vi "Two Camera.vi"() -> ()   [LabVIEW 2015]
uses:
  <vilib>/userdefined/High Color/IMAQdx.ctl
  <vilib>/vision/driver/NI_Vision_Acquisition_Software.lvlib
panel:
  in  "Save":bool
  in  "Session In 2":T1
  in  "Session In":T1
  out "Image 2":T2(plugin-control)
  out "Frame Rate 2":dbl=6.261180679785331 caption="Frame Rate"
  out "Image Number 2":u32=152 caption="Image Number"
  in  "File Name 2":string
  in  "Path 2":path=path "C:/Users/PKU210/Desktop/SavePicture" caption="Images Folder"
  in  "Path":path=path "C:/Users/PKU210/Desktop/SavePicture" caption="Images Folder"
  in  "File Name":string
  out "Image Number":u32=152
  out "Frame Rate":dbl=6.261180679785331
  in  "Stop":bool
  out "Image":T2(plugin-control)
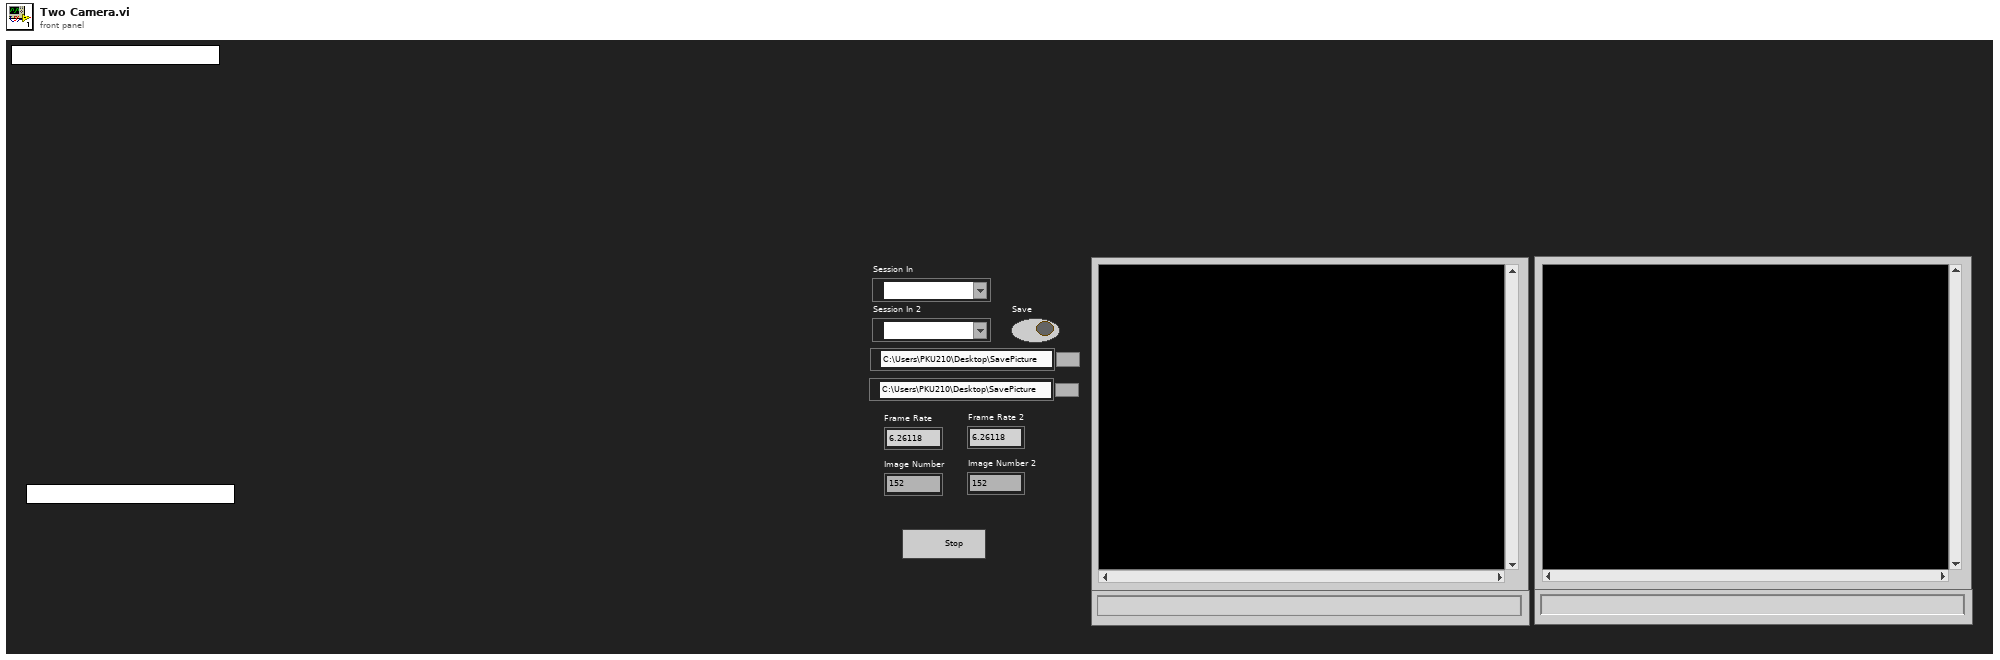
[diagram p1: front panel]
types:
  T1 = typedef "IMAQdx.ctl" = refnum<k21>
  T2 = typedef "IMAQ Image.ctl" = refnum<image>
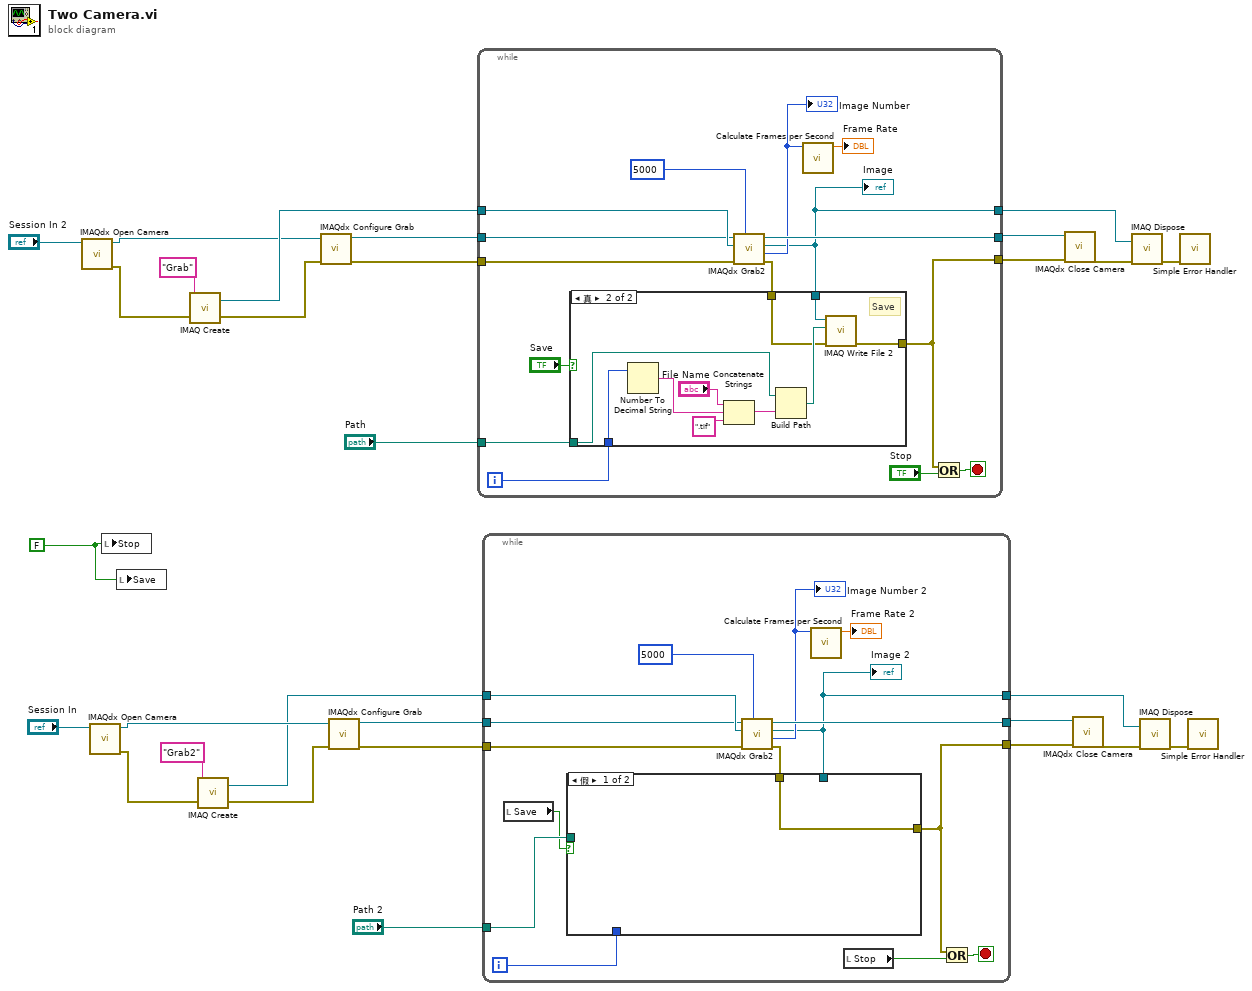
[diagram p0: block diagram]
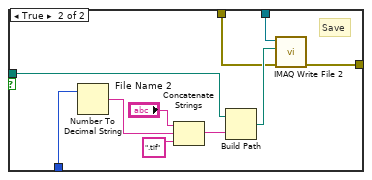
[diagram p2: hidden frame]
diagram:
  w1 = FALSE ("Stop")
  n1 = call <vilib>:"IMAQdx Open Camera.vi"("Session In"="Session In 2") -> ("error out"=w25:errorcluster, "Session Out"=w24:T1)  [unwired: 9 in]
  n2 = call <vilib>:"IMAQdx Open Camera.vi"("Session In"="Session In") -> ("error out"=w8:errorcluster, "Session Out"=w9:T1)  [unwired: 9 in]
  n3 = local write "Stop"(w1) -> ()
  n4 = local write "Save"(w1) -> ()
  n5 = call "IMAQ Create"("Image Name"="Grab", "error in (no error)"=w25) -> ("New Image"=w29:T2, "error out"=w18:errorcluster)  [unwired: 2 in, 1 out]
  n6 = call "IMAQ Create"("Image Name"="Grab2", "error in (no error)"=w8) -> ("New Image"=w4:T2, "error out"=w15:errorcluster)  [unwired: 2 in, 1 out]
  n7 = call <vilib>:"IMAQdx Configure Grab.vi"("error in"=w18, "Session In"=w24) -> ("error out"=w20:errorcluster, "Session Out"=w23:T1)  [unwired: 8 in]
  n8 = call <vilib>:"IMAQdx Configure Grab.vi"("error in"=w15, "Session In"=w9) -> ("error out"=w13:errorcluster, "Session Out"=w10:T1)  [unwired: 8 in]
  n9 = while {
    tunnel: [w41] -> w22
    tunnel: w29 -> [w42]
    tunnel: w20 -> [w37]
    tunnel: [w33] -> w28
    tunnel: w23 -> [w38]
    tunnel: [w31] -> w19
    tunnel: "Path" -> [w35]
    i -> [w34]
    stop <- w44 stop-if-true
    n10 = call <vilib>:"IMAQdx Grab2.vi"("Timeout (ms)"=5000, "error in"=w37, "Image In"=w42, "Session In"=w38) -> ("error out"=w32:errorcluster, "Buffer Number Out"=w39:u32, "Image Out"=w33:T2, "Session Out"=w41:T1)  [unwired: 4 in]
    "Image" <- w33
    "Image Number" <- w39
    n11 = case shown="真" "Save" {
      tunnel: w35 -> [_ w50]
      tunnel: w34 -> [_ w49]
      tunnel: w33 -> [_ w48]
      tunnel: w32 -> [w45 w47]
      tunnel: [w45 w46] -> w31
      frame False {
      }
      frame True {
        # "Save"
        n12 = Number To Decimal String(number=w49) -> (decimal integer string=w52:string)  [unwired: 1 in]
        n13 = Concatenate Strings("File Name", w52, ".tif" ("字符串")) -> (w51:string)
        n14 = Build Path(base path=w50, name or relative path=w51) -> (appended path=w54:path)
        n15 = call-poly "IMAQ Write File 2"("error in (no error)"=w47, "File Path"=w54, "Image"=w48) -> ("error out"=w46:errorcluster)  [unwired: 7 in, 1 out]
      }
    }
    n16 = call <vilib>:"Calculate Frames per Second.vi"("Buffer Number"=w39) -> ("Acquired Frames/s"=→"Frame Rate":dbl)  [unwired: 2 in, 8 out]
    n17 = Or(x=w31, y="Stop") -> (x .or. y?=w44:bool)
  }
  n18 = while {
    tunnel: [w68] -> w11
    tunnel: w4 -> [w69]
    tunnel: w13 -> [w64]
    tunnel: [w60] -> w5
    tunnel: w10 -> [w65]
    tunnel: [w58] -> w14
    tunnel: "Path 2" -> [w62]
    i -> [w61]
    stop <- w70 stop-if-true
    n19 = local read "Save"() -> (w56:bool)
    n20 = call <vilib>:"IMAQdx Grab2.vi"("Timeout (ms)"=5000, "error in"=w64, "Image In"=w69, "Session In"=w65) -> ("error out"=w59:errorcluster, "Buffer Number Out"=w66:u32, "Image Out"=w60:T2, "Session Out"=w68:T1)  [unwired: 4 in]
    "Image 2" <- w60
    "Image Number 2" <- w66
    n21 = case shown="假" w56 {
      tunnel: w62 -> [_ w76]
      tunnel: w61 -> [_ w75]
      tunnel: w60 -> [_ w74]
      tunnel: w59 -> [w71 w73]
      tunnel: [w71 w72] -> w58
      frame False {
      }
      frame True {
        # "Save"
        n22 = Number To Decimal String(number=w75) -> (decimal integer string=w78:string)  [unwired: 1 in]
        n23 = Concatenate Strings("File Name 2", w78, ".tif" ("字符串")) -> (w77:string)
        n24 = Build Path(base path=w76, name or relative path=w77) -> (appended path=w80:path)
        n25 = call-poly "IMAQ Write File 2"("error in (no error)"=w73, "File Path"=w80, "Image"=w74) -> ("error out"=w72:errorcluster)  [unwired: 7 in, 1 out]
      }
    }
    n26 = call <vilib>:"Calculate Frames per Second.vi"("Buffer Number"=w66) -> ("Acquired Frames/s"=→"Frame Rate 2":dbl)  [unwired: 2 in, 8 out]
    n27 = local read "Stop"() -> (w57:bool)
    n28 = Or(x=w58, y=w57) -> (x .or. y?=w70:bool)
  }
  n29 = call <vilib>:"IMAQdx Close Camera.vi"("error in"=w19, "Session In"=w22) -> ("error out"=w21:errorcluster)  [unwired: 9 in]
  n30 = call <vilib>:"IMAQdx Close Camera.vi"("error in"=w14, "Session In"=w11) -> ("error out"=w12:errorcluster)  [unwired: 9 in]
  n31 = call "IMAQ Dispose"("Image"=w28, "error in (no error)"=w21) -> ("error out"=w27:errorcluster)  [unwired: 1 in, 3 out]
  n32 = call "IMAQ Dispose"("Image"=w5, "error in (no error)"=w12) -> ("error out"=w6:errorcluster)  [unwired: 1 in, 3 out]
  n33 = call <vilib>:"Simple Error Handler.vi"("error in (no error)"=w27) -> ()  [unwired: 1 in, 8 out]
  n34 = call <vilib>:"Simple Error Handler.vi"("error in (no error)"=w6) -> ()  [unwired: 1 in, 8 out]
